vi "butterfly valve control.vi"() -> ()   [LabVIEW 2013]
uses:
  <vilib>/Instr/_visa.llb/VISA Configure Serial Port (Instr).vi
panel:
  in  "Vertical Pointer Slide":dbl(slide) scale=0.0..100.0
  in  "Valve Position (% Opened)":dbl min=0.0 max=100.0 step=5.0
  in  "O/C":bool
  out "read buffer 4":string
  out "read buffer":string
  out "Valve position (%)":dbl
  out "Pressure (Torr)":dbl(graph)
  in  "Butterfly Valve":T1(radio)
  in  "stop":bool
  out "error out":errorcluster
  out "Meter":dbl(knob) scale=0.0..100.0
  # "M106"
  # "T40"
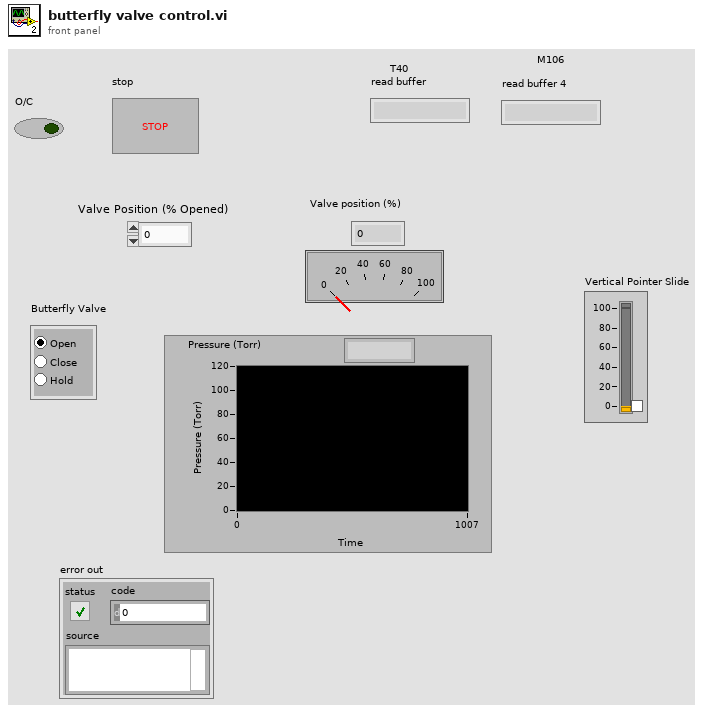
[diagram p1: front panel]
types:
  T1 = enum32{" Selection 1", "Radio Selection 2", "RadioSelection 4"}
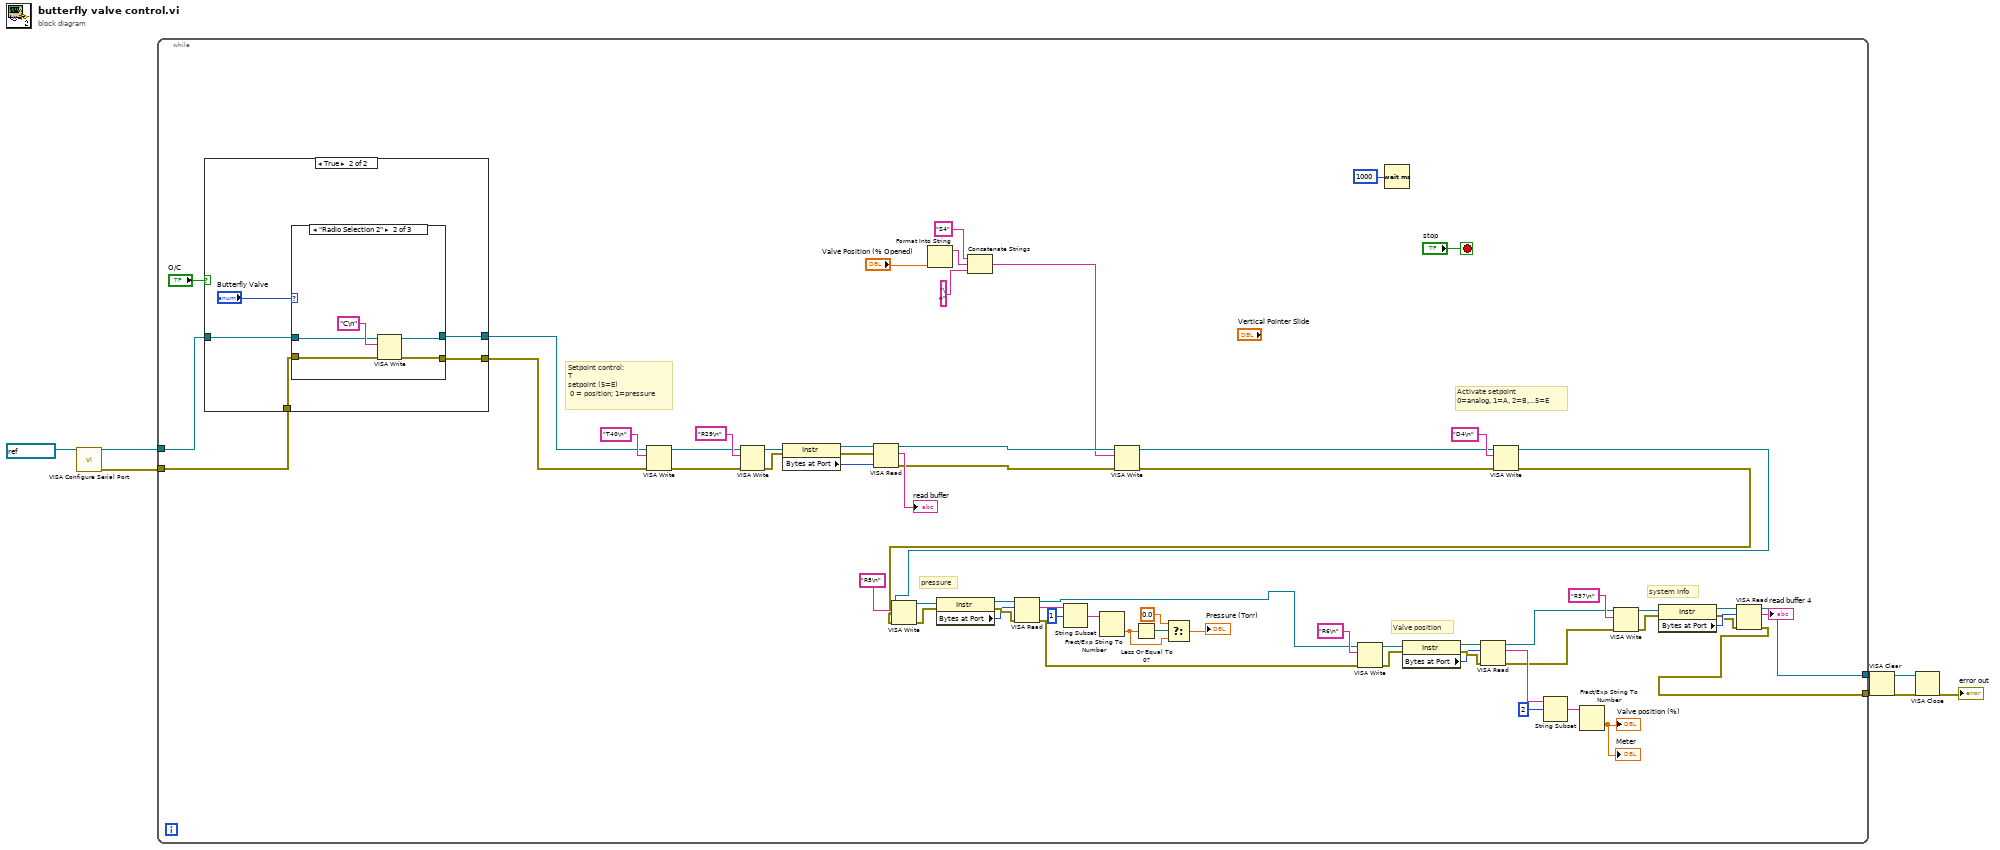
[diagram p0: block diagram]
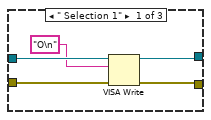
[diagram p3: hidden frame]
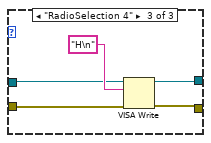
[diagram p4: hidden frame]
diagram:
  n1 = call-poly "VISA Configure Serial Port"("VISA resource name"=refnum<visa-resource-name> "COM5") -> ("VISA resource name out"=w7:refnum<visa-resource-name>, "error out"=w3:errorcluster)  [unwired: 13 in]
  n2 = while {
    tunnel: w7 -> [w18]
    tunnel: w3 -> [w15]
    tunnel: [w27] -> w2
    tunnel: [w26] -> w1
    stop <- "stop" stop-if-true
    # "system info"
    # "Activate setpoint \n0=analog, 1=A, 2=B,...5=E"
    # "pressure"
    # "Valve position"
    # "Setpoint control:\nT\nsetpoint (5=E)\n 0 = position; 1=pressure"
    n3 = case shown="True" "O/C" {
      tunnel: w18 -> [w75 w79]
      tunnel: [w75 w78] -> w17
      tunnel: [w74 w77] -> w16
      tunnel: w15 -> [w74 w76]
      frame False {
      }
      frame True {
        n4 = case shown="\"Radio Selection 2\"" "Butterfly Valve" {
          tunnel: w79 -> [w85 w89 w92]
          tunnel: [w83 w88 w94] -> w78
          tunnel: w76 -> [w82 w87 w91]
          tunnel: [w81 w86 w93] -> w77
          frame " Selection 1" {
            n5 = VISA Write(VISA resource name=w85, write buffer="O\n", error in (no error)=w82) -> (VISA resource name out=w83:refnum<visa-resource-name>, error out=w81:errorcluster)  [unwired: 1 out]
          }
          frame "Radio Selection 2" {
            n6 = VISA Write(VISA resource name=w89, write buffer="C\n", error in (no error)=w87) -> (VISA resource name out=w88:refnum<visa-resource-name>, error out=w86:errorcluster)  [unwired: 1 out]
          }
          frame "RadioSelection 4" {
            n7 = VISA Write(VISA resource name=w92, write buffer="H\n", error in (no error)=w91) -> (VISA resource name out=w94:refnum<visa-resource-name>, error out=w93:errorcluster)  [unwired: 1 out]
          }
        }
      }
    }
    n8 = VISA Write(VISA resource name=w17, write buffer="T40\n", error in (no error)=w16) -> (VISA resource name out=w23:refnum<visa-resource-name>, error out=w38:errorcluster)  [unwired: 1 out]
    n9 = VISA Write(VISA resource name=w23, write buffer="R29\n", error in (no error)=w38) -> (VISA resource name out=w44:refnum<visa-resource-name>, error out=w43:errorcluster)  [unwired: 1 out]
    n10 = property class="Instr"(reference=w44, error in=w43) -> (reference out=w46:refnum<visa-resource-name>, error out=w45:errorcluster, "Bytes at Port"=w24:u32)
    n11 = VISA Read(VISA resource name=w46, byte count=w24, error in (no error)=w45) -> (VISA resource name out=w39:refnum<visa-resource-name>, read buffer=→"read buffer":string, error out=w40:errorcluster)  [unwired: 1 out]
    n12 = Format Into String("Valve Position (% Opened)") -> (resulting string=w9:string)  [unwired: 3 in, 1 out]
    n13 = Concatenate Strings("S4" ("string"), w9, "\n" ("string")) -> (w12:string)
    n14 = VISA Write(VISA resource name=w39, write buffer=w12, error in (no error)=w40) -> (VISA resource name out=w21:refnum<visa-resource-name>, error out=w22:errorcluster)  [unwired: 1 out]
    n15 = Wait (ms)(milliseconds to wait=u32 1000) -> ()  [unwired: 1 out]
    n16 = VISA Write(VISA resource name=w21, write buffer="D4\n", error in (no error)=w22) -> (VISA resource name out=w20:refnum<visa-resource-name>, error out=w19:errorcluster)  [unwired: 1 out]
    n17 = VISA Write(VISA resource name=w20, write buffer="R5\n", error in (no error)=w19) -> (VISA resource name out=w59:refnum<visa-resource-name>, error out=w58:errorcluster)  [unwired: 1 out]
    n18 = property class="Instr"(reference=w59, error in=w58) -> (reference out=w62:refnum<visa-resource-name>, error out=w61:errorcluster, "Bytes at Port"=w60:u32)
    n19 = VISA Read(VISA resource name=w62, byte count=w60, error in (no error)=w61) -> (VISA resource name out=w37:refnum<visa-resource-name>, read buffer=w55:string, error out=w36:errorcluster)  [unwired: 1 out]
    n20 = String Subset(string=w55, offset (0)=1) -> (substring=w57:string)  [unwired: 1 in]
    n21 = Fract/Exp String To Number(string=w57) -> (number=w49:dbl)  [unwired: 3 in, 1 out]
    n22 = Less Or Equal To 0?(x=w49) -> (x <= 0?=w52:bool)
    n23 = Select(t=0.0, s=w52, f=w49) -> (s? t:f=→"Pressure (Torr)":dbl)
    n24 = VISA Write(VISA resource name=w37, write buffer="R6\n", error in (no error)=w36) -> (VISA resource name out=w68:refnum<visa-resource-name>, error out=w67:errorcluster)  [unwired: 1 out]
    n25 = property class="Instr"(reference=w68, error in=w67) -> (reference out=w71:refnum<visa-resource-name>, error out=w70:errorcluster, "Bytes at Port"=w69:u32)
    n26 = VISA Read(VISA resource name=w71, byte count=w69, error in (no error)=w70) -> (VISA resource name out=w29:refnum<visa-resource-name>, read buffer=w66:string, error out=w28:errorcluster)  [unwired: 1 out]
    n27 = String Subset(string=w66, offset (0)=2) -> (substring=w64:string)  [unwired: 1 in]
    n28 = Fract/Exp String To Number(string=w64) -> (number=→"Valve position (%)" →"Meter":dbl)  [unwired: 3 in, 1 out]
    n29 = VISA Write(VISA resource name=w29, write buffer="R37\n", error in (no error)=w28) -> (VISA resource name out=w34:refnum<visa-resource-name>, error out=w35:errorcluster)  [unwired: 1 out]
    n30 = property class="Instr"(reference=w34, error in=w35) -> (reference out=w31:refnum<visa-resource-name>, error out=w32:errorcluster, "Bytes at Port"=w33:u32)
    n31 = VISA Read(VISA resource name=w31, byte count=w33, error in (no error)=w32) -> (VISA resource name out=w26:refnum<visa-resource-name>, read buffer=→"read buffer 4":string, error out=w27:errorcluster)  [unwired: 1 out]
  }
  n32 = VISA Clear(VISA resource name=w1, error in (no error)=w2) -> (VISA resource name out=w6:refnum<visa-resource-name>, error out=w5:errorcluster)
  n33 = VISA Close(VISA resource name=w6, error in (no error)=w5) -> (error out=→"error out":errorcluster)
